vi "Move Core.vi"(6 "Relative?":bool, 8 "error in (no error)":errorcluster, 9 "Raw-Position":dbl, 10 "AxisNumber":u8, 11 "CS++SimMotor in":refnum<class "CS++SimMotor.lvclass">) -> (0 "error out":errorcluster, 3 "CS++SimMotor out":refnum<class "CS++SimMotor.lvclass">)   [LabVIEW 2015, in "CS++SimMotor.lvlib" / "CS++SimMotor.lvclass"]
doc: "Starts an absolute or relative movment of an axis."
uses:
  CS++SimMotor.lvclass
  CS++SimMotor.lvclass/CS++SimMotor.ctl
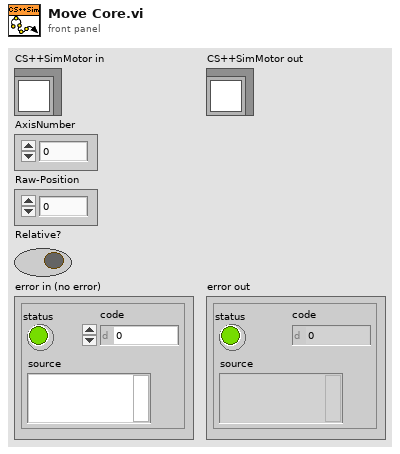
[diagram p1: front panel]
types:
  T1 = enum16{"RelativeMovement", "AbsoluteMovement", "Stop", "ReferenceMovement"}
  T2 = cluster{"AxisNumber":u8, "Raw-Position":dbl, "Enum":enum16{"RelativeMovement", "AbsoluteMovement", "Stop", "ReferenceMovement"}}
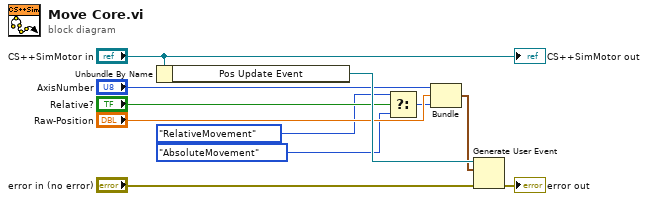
[diagram p0: block diagram]
diagram:
  n1 = Unbundle By Name("CS++SimMotor in") -> ("Pos Update Event"=w11:refnum<user-event>)
  n2 = Select(t=T1."RelativeMovement" ("Enum"), s="Relative?", f=T1."AbsoluteMovement" ("Enum")) -> (s? t:f=w2:T1)
  n3 = Bundle("AxisNumber"="AxisNumber", "Raw-Position"="Raw-Position", "Enum"=w2) -> (w8:T2)  [unwired: 1 in]
  n4 = Generate User Event(user event=w11, event data cluster=w8, error in="error in (no error)") -> (error out=→"error out":errorcluster)  [unwired: 1 in, 1 out]
  "CS++SimMotor out" <- "CS++SimMotor in"
